vi "Subset Buffers.vi"(6 "inline buffer offset":u64 format="%d bytes", 7 "string buffer offset":u64 format="%d bytes", 8 "error in (no error)":errorcluster, 9 "inline buffer size":u64 format="%d bytes", 10 "string buffer size":u64 format="%d bytes", 11 "Buffers in":refnum<class "Buffers.lvclass">) -> (0 "error out":errorcluster, 2 "subset Buffers":refnum<class "Buffers.lvclass">, 3 "Buffers out":refnum<class "Buffers.lvclass">, 4 "inline buffer offset +size":u64 format="%d bytes", 5 "string buffer offset + size":u64 format="%d bytes")   [LabVIEW 2017, in "DSF Core.lvlib" / "Buffers.lvclass"]
uses:
  Buffers.lvclass
  Buffers.lvclass/Buffers.ctl
  Buffer.lvclass
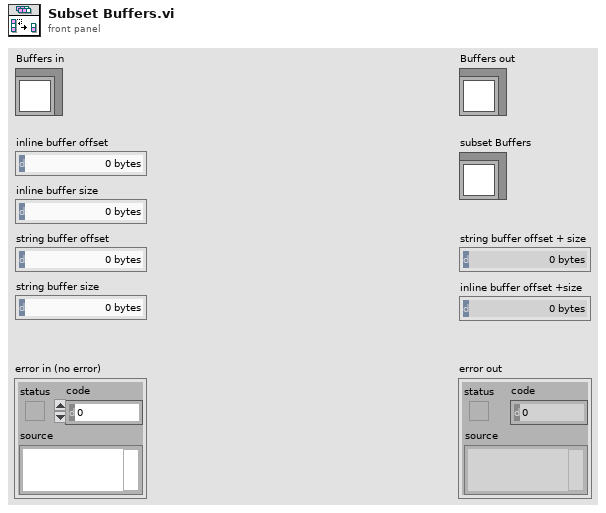
[diagram p1: front panel]
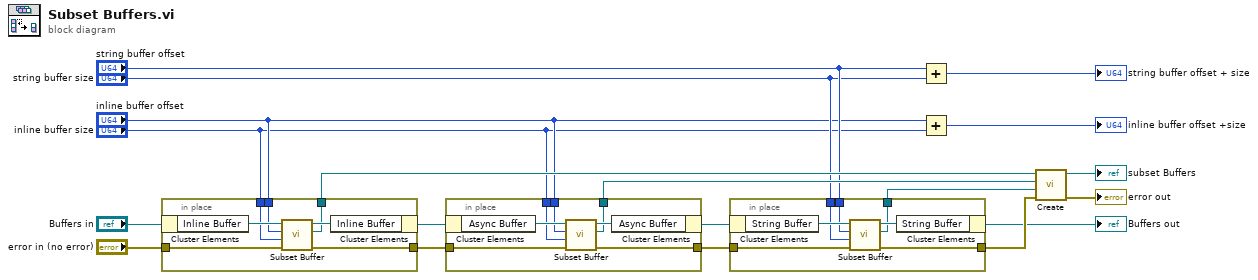
[diagram p0: block diagram]
diagram:
  n1 = in-place {
    in-place-border: "error in (no error)" -> [w24]
    in-place-border: [w23] -> w15
    in-place-border: "inline buffer offset" -> [w22]
    in-place-border: "inline buffer size" -> [w21]
    in-place-border: [w20] -> w8
    n2 = in-place-cluster #1("Buffers in") -> ("Inline Buffer"=w26:refnum<class "Buffer.lvclass">)
    n3 = call "Subset Buffer.vi"("error in (no error)"=w24, "size"=w21, "offset"=w22, "Buffer in"=w26) -> ("error out"=w23:errorcluster, "subset Buffer"=w20:refnum<class "Buffer.lvclass">, "Buffer out"=w25:refnum<class "Buffer.lvclass">)  [unwired: 4 in, 1 out]
    n4 = in-place-cluster #1("Inline Buffer"=w25) -> (w14:refnum<class "Buffers.lvclass">)
  }
  n5 = in-place {
    in-place-border: w15 -> [w31]
    in-place-border: [w30] -> w12
    in-place-border: "inline buffer offset" -> [w29]
    in-place-border: "inline buffer size" -> [w28]
    in-place-border: [w27] -> w9
    n6 = in-place-cluster #2(w14) -> ("Async Buffer"=w33:refnum<class "Buffer.lvclass">)
    n7 = call "Subset Buffer.vi"("error in (no error)"=w31, "size"=w28, "offset"=w29, "Buffer in"=w33) -> ("error out"=w30:errorcluster, "subset Buffer"=w27:refnum<class "Buffer.lvclass">, "Buffer out"=w32:refnum<class "Buffer.lvclass">)  [unwired: 4 in, 1 out]
    n8 = in-place-cluster #2("Async Buffer"=w32) -> (w13:refnum<class "Buffers.lvclass">)
  }
  n9 = in-place {
    in-place-border: w12 -> [w38]
    in-place-border: [w37] -> w11
    in-place-border: "string buffer offset" -> [w35]
    in-place-border: "string buffer size" -> [w36]
    in-place-border: [w34] -> w10
    n10 = in-place-cluster #3(w13) -> ("String Buffer"=w40:refnum<class "Buffer.lvclass">)
    n11 = call "Subset Buffer.vi"("error in (no error)"=w38, "size"=w36, "offset"=w35, "Buffer in"=w40) -> ("error out"=w37:errorcluster, "subset Buffer"=w34:refnum<class "Buffer.lvclass">, "Buffer out"=w39:refnum<class "Buffer.lvclass">)  [unwired: 4 in, 1 out]
    n12 = in-place-cluster #3("String Buffer"=w39) -> (→"Buffers out":refnum<class "Buffers.lvclass">)
  }
  n13 = Add(x="string buffer offset", y="string buffer size") -> (x+y=→"string buffer offset + size":u64)
  n14 = Add(x="inline buffer offset", y="inline buffer size") -> (x+y=→"inline buffer offset +size":u64)
  n15 = call "Create.vi"("error in (no error)"=w11, "String Buffer (null)"=w10, "Async Buffer (null)"=w9, "Inline Buffer (null)"=w8) -> ("error out"=→"error out":errorcluster, "Buffers out"=→"subset Buffers":refnum<class "Buffers.lvclass">)  [unwired: 6 in]
